vi "Identities.vi"(8 "error in (no error)":errorcluster, 11 "EventAPI in":refnum<class "EventAPI.lvclass">) -> (0 "error out":errorcluster, 2 "Identities":refnum<class "Identity.lvclass">[](array[class]), 3 "EventAPI out":refnum<class "EventAPI.lvclass">)   [LabVIEW 2020, in "Volatus.lvlib" / "EventAPI.lvclass"]
uses:
  EventAPI.lvclass
  EventAPI.lvclass/EventAPI.ctl
  ApiIdentity/ApiIdentity.lvclass
  C:/dev/lv20CE/relink/lv-volatus/Volatus/ApiIdentity/ApiIdentity.lvclass
  C:/dev/lv20CE/relink/lv-volatus/Volatus/Identity/Identity.lvclass
  Identity/Identity.lvclass
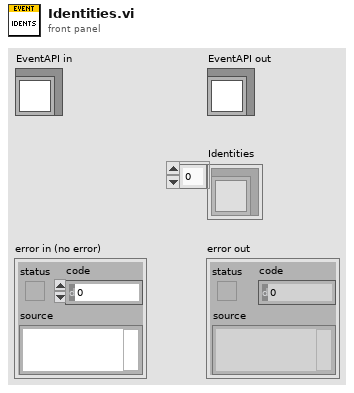
[diagram p1: front panel]
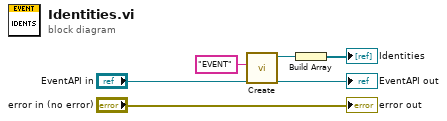
[diagram p0: block diagram]
diagram:
  n1 = call "Create.vi"("API ID"="EVENT") -> ("ApiIdentity out"=w2:refnum<class "ApiIdentity.lvclass">)  [unwired: 10 in]
  n2 = Build Array(w2) -> (→"Identities":refnum<class "ApiIdentity.lvclass">[])
  "error out" <- "error in (no error)"
  "EventAPI out" <- "EventAPI in"
